vi "Warnings.vi"() -> (3 "project name":string, 4 "invalid project path":string, 6 "incompatible project version":string, 8 "invalid measurement path":string, 10 "incompatible measurement version":string, 13 "permission error":string, 14 "invalid folder/file names":string, 15 "drive selection":string)   [LabVIEW 2021, in "Converter.lvlib"]
uses:
  Converter.lvlib
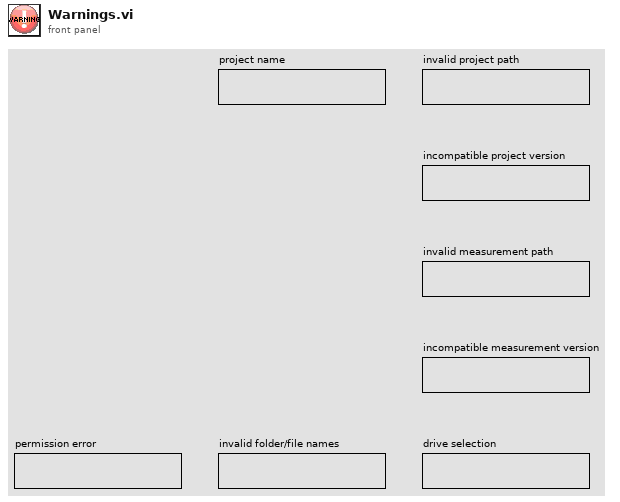
[diagram p1: front panel]
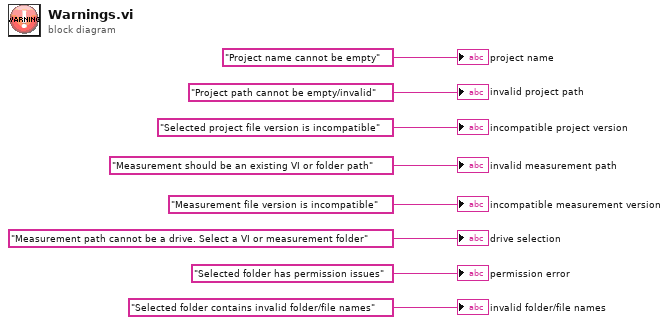
[diagram p0: block diagram]
diagram:
  "invalid project path" <- "Project path cannot be empty/invalid" ("Invalid project path")
  "incompatible project version" <- "Selected project file version is incompatible" ("Invalid project path")
  "invalid measurement path" <- "Measurement should be an existing VI or folder path" ("Invalid project path")
  "incompatible measurement version" <- "Measurement file version is incompatible" ("Invalid project path")
  "drive selection" <- "Measurement path cannot be a drive. Select a VI or measurement folder" ("Invalid project path")
  "project name" <- "Project name cannot be empty" ("Project name")
  "permission error" <- "Selected folder has permission issues" ("Invalid project path")
  "invalid folder/file names" <- "Selected folder contains invalid folder/file names" ("Invalid project path")
